vi "Global.vi"() -> ()   [LabVIEW 2023]
panel:
  in  "ValChange":T1(ring)
  out "ValChange 4":bool
  out "ValChange 3":bool
  out "ValChange 2":bool
  out "ValChange 1":bool
  out "Sema":T2
  out "ATmega328":refnum<visa-resource-name>
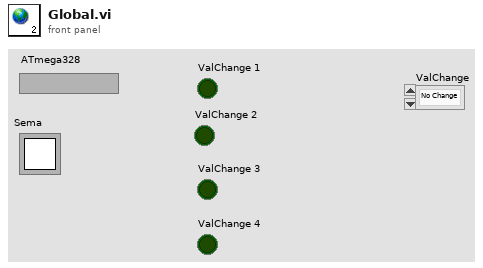
[diagram p1: front panel]
types:
  T1 = enum16{"No Change", "Serv 1", "Serv 2", "Serv 3", "Serv 4"}
  T2 = typedef "Semaphore RefNum" = refnum<k1>
diagram:
